vi "RichToFlatnixnet_grpc_ConvertFramesToSignalsSinglePointResponse.vi"(5 "OutputClusterType":T1, 11 "InputCluster":T2) -> (3 "OutputCluster":T1)   [LabVIEW 2025, in "xnet-grpc_client.lvlib"]
uses:
  nixnet_grpc_ConvertFramesToSignalsSinglePointResponse.ctl
  nixnet_grpc_ConvertFramesToSignalsSinglePointResponse_Flat.ctl
  xnet-grpc_client.lvlib
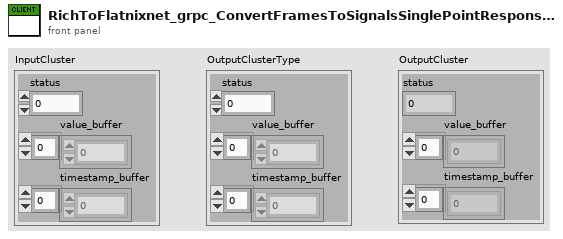
[diagram p1: front panel]
types:
  T1 = typedef "xnet-grpc_client.lvlib/nixnet_grpc_ConvertFramesToSignalsSinglePointResponse_Flat.ctl" = cluster{"status":i32, "value_buffer":dbl[], "timestamp_buffer":u64[]}
  T2 = typedef "xnet-grpc_client.lvlib/nixnet_grpc_ConvertFramesToSignalsSinglePointResponse.ctl" = cluster{"status":i32, "value_buffer":dbl[], "timestamp_buffer":u64[]}
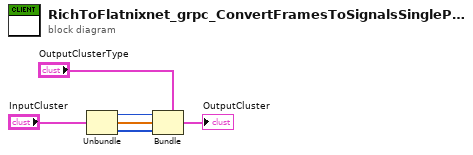
[diagram p0: block diagram]
diagram:
  n1 = Unbundle "Unbundle"("InputCluster") -> ("status"=w3:i32, "value_buffer"=w2:dbl[], "timestamp_buffer"=w1:u64[])
  n2 = Bundle "Bundle"(cluster="OutputClusterType", "status"=w3, "value_buffer"=w2, "timestamp_buffer"=w1) -> (→"OutputCluster":T1)
